vi "Scan for Motors.vi"(7 "Search Timeout (10000 ms)":u32=10000, 8 "error in (no error)":errorcluster, 9 "Ending ID (253)":u8=253, 10 "Starting ID (0)":u8, 11 "Dynamixel Motor VISA in":refnum<class "Dynamixel Motor VISA.lvclass">) -> (0 "error out":errorcluster, 2 "Motors IDs Found":u8[](array[numeric]), 3 "Dynamixel Motor VISA out":refnum<class "Dynamixel Motor VISA.lvclass">)   [LabVIEW 2016, in "Dynamixel Motor VISA.lvclass"]
doc: "Scans sequentially for motors between <b>Starting ID</b> and <b>Ending ID</b> for no longer than <b>Search Timeout</b>. If all of the motors do not have unique IDs, then motors with duplicate IDs may not be found."
uses:
  <instrlib>/Dynamixel Motor/HAIOL/VISA/Dynamixel Motor VISA.lvclass
  <instrlib>/Dynamixel Motor/HAIOL/VISA/Dynamixel Motor VISA.lvclass/Dynamixel Motor VISA.ctl
  <instrlib>/Dynamixel Motor/Dynamixel Motor.lvlib
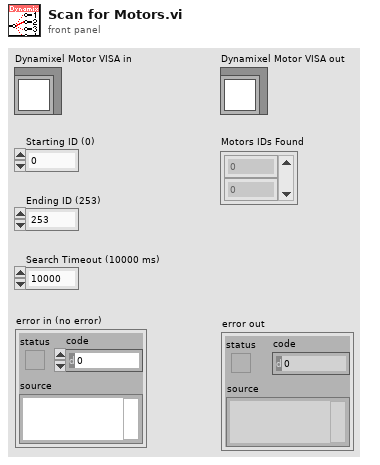
[diagram p1: front panel]
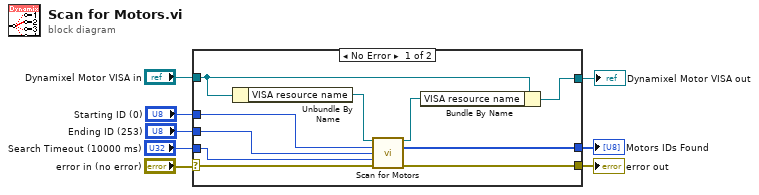
[diagram p0: block diagram]
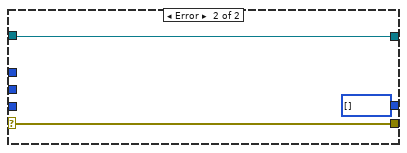
[diagram p2: hidden frame]
diagram:
  n1 = case shown="No Error" "error in (no error)" {
    selector: "error in (no error)" -> [w18 w19]
    tunnel: "Dynamixel Motor VISA in" -> [w11 w21]
    tunnel: "Starting ID (0)" -> [w16 _]
    tunnel: "Ending ID (253)" -> [w15 _]
    tunnel: "Search Timeout (10000 ms)" -> [w14 _]
    tunnel: [w13 w19] -> w3
    tunnel: [w12 u8[] [] ("Motors IDs Found")] -> w2
    tunnel: [w9 w21] -> w1
    frame No Error {
      n2 = Unbundle By Name(w11) -> ("VISA resource name"=w17:refnum<visa-resource-name>)
      n3 = call <instrlib>:"Scan for Motors.vi"("VISA resource name"=w17, "Starting ID (0)"=w16, "Ending ID (253)"=w15, "Search Timeout (10000 ms)"=w14, "error in (no error)"=w18) -> ("VISA resource name out"=w10:refnum<visa-resource-name>, "Motors IDs Found"=w12:u8[], "error out"=w13:errorcluster)  [unwired: 8 in]
      n4 = Bundle By Name(cluster=w11, "VISA resource name"=w10) -> (w9:refnum<class "Dynamixel Motor VISA.lvclass">)
    }
    frame Error {
    }
  }
  "error out" <- w3
  "Dynamixel Motor VISA out" <- w1
  "Motors IDs Found" <- w2
